vi "ConfigureFlowUnit.vi"(0 "object in":refnum<class "CetoniPump.lvclass">, 1 "index":i32, 2 "FlowUnits":T4={"Prefix"=-3, "TimeUnit"=60, "VolumeUnit"=68} {"VolumeUnit" items=["LITRES"=68]; "TimeUnit" items=["PER_SECOND"=1, "PER_MINUTE"=60, "PER_HOUR"=3600]; "Prefix" items=["UNIT"=0, "DECI"=-1, "CENTI"=-2, "MILLI"=-3, "MICRO"=-6]}, 5 "error in (no error)":errorcluster) -> (14 "object out":refnum<class "CetoniPump.lvclass">, 19 "error out":errorcluster)   [LabVIEW 2021, in "CetoniPump.lvclass"]
uses:
  CetoniPump.lvclass
  CetoniPump.lvclass/CetoniPump.ctl
  Users/olaja/AppData/Local/CETONI_SDK/lib/labview/labbCAN_Pump_API/labbCAN_Pump_API.lvlib
  Users/olaja/AppData/Local/CETONI_SDK/lib/labview/labbCAN_Bus_API/SiUnitPrefix.ctl
  Users/olaja/AppData/Local/CETONI_SDK/lib/labview/labbCAN_Bus_API/labbCAN_Bus_API.lvlib
  Users/olaja/AppData/Local/CETONI_SDK/lib/labview/labbCAN_Bus_API/TimeUnits.ctl
  Users/olaja/AppData/Local/CETONI_SDK/lib/labview/labbCAN_Pump_API/VolumeUnits.ctl
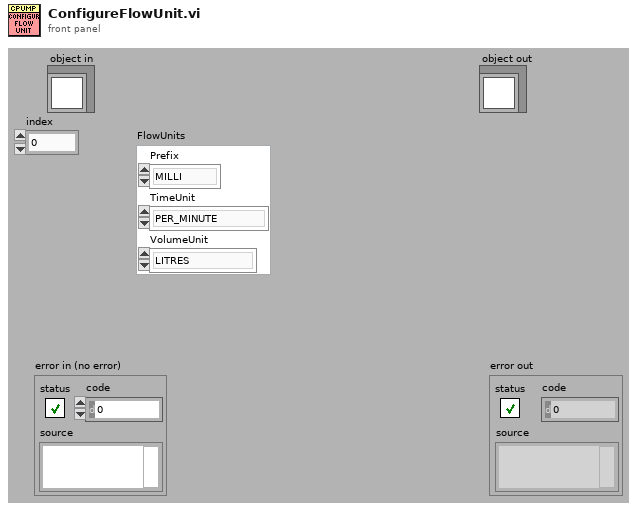
[diagram p1: front panel]
types:
  T1 = typedef "labbCAN_Bus_API.lvlib/SiUnitPrefix.ctl" = i32
  T2 = typedef "labbCAN_Bus_API.lvlib/TimeUnits.ctl" = i32
  T3 = typedef "labbCAN_Pump_API.lvlib/VolumeUnits.ctl" = i32
  T4 = cluster{"Prefix":T1, "TimeUnit":T2, "VolumeUnit":T3}
  T5 = cluster{"Pump Handle":i64, "Pump Name":string, "Maximum Volume":dbl, "Maximum Flow Rate":dbl, "Flow Rate":dbl, "Fill Level":dbl}[]
  T6 = cluster{"Pump Handle":i64, "Pump Name":string, "Maximum Volume":dbl, "Maximum Flow Rate":dbl, "Flow Rate":dbl, "Fill Level":dbl}
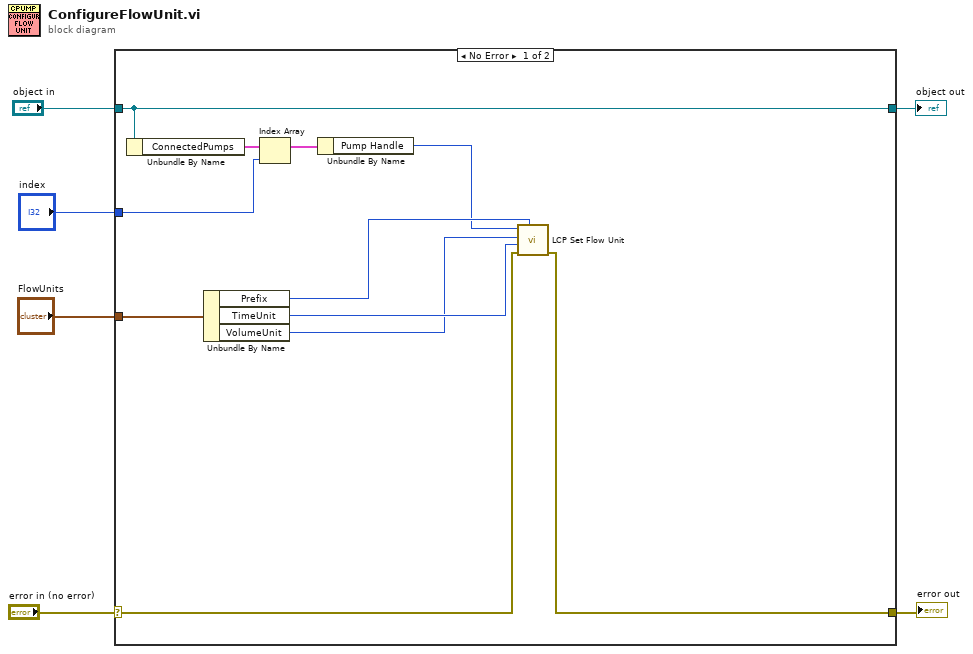
[diagram p0: block diagram]
diagram:
  n1 = case shown="No Error" "error in (no error)" {
    selector: "error in (no error)" -> [w11 w19]
    tunnel: [w10 w19] -> w5
    tunnel: [w17 w18] -> w3
    tunnel: "object in" -> [w17 w18]
    tunnel: "FlowUnits" -> [w15 _]
    tunnel: "index" -> [w8 _]
    frame No Error {
      n2 = Unbundle By Name(w17) -> ("ConnectedPumps"=w16:T5)
      n3 = Unbundle By Name(w15) -> ("Prefix"=w14:T1, "TimeUnit"=w13:T2, "VolumeUnit"=w12:T3)
      n4 = Index Array(array=w16, index=w8) -> (element=w9:T6)
      n5 = Unbundle By Name(w9) -> ("Pump Handle"=w7:i64)
      n6 = call "LCP Set Flow Unit.vi"("Prefix"=w14, "error in (no error)"=w11, "TimeUnit"=w13, "VolumeUnit"=w12, "Pump Handle"=w7) -> ("error out"=w10:errorcluster)  [unwired: 6 in]
    }
    frame Error {
    }
  }
  "error out" <- w5
  "object out" <- w3
